vi "1D_2Period.vi"(1 "delt":dbl, 2 "1Darray":dbl[](array[numeric])) -> (0 "T2":dbl)   [LabVIEW 2020]
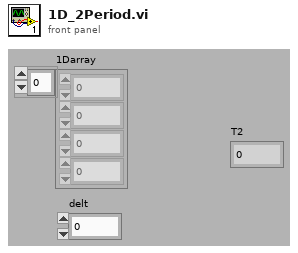
[diagram p1: front panel]
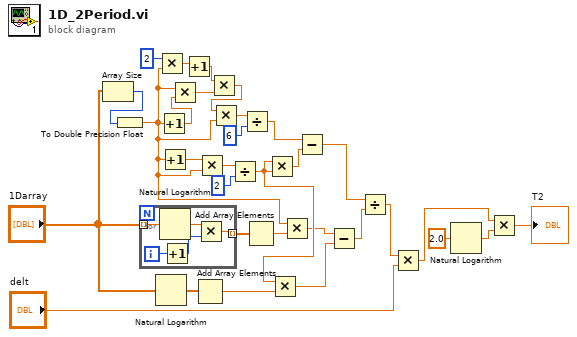
[diagram p0: block diagram]
diagram:
  n1 = Array Size(array="1Darray") -> (size(s)=w8:i32)
  n2 = To Double Precision Float(number=w8) -> (double precision float=w7:dbl)
  n3 = for {
    tunnel: "1Darray" -> [w36] mode=indexing
    tunnel: [w32] -> w21 mode=indexing
    i -> [w35]
    n4 = Natural Logarithm(1:w36) -> (0:w34:dbl)
    n5 = Increment(x=w35) -> (x+1=w33:i32)
    n6 = Multiply(x=w34, y=w33) -> (x*y=w32:dbl)
  }
  n7 = Natural Logarithm(1:"1Darray") -> (0:w16:dbl[])
  n8 = Multiply(x=2 ("count"), y=w7) -> (x*y=w28:dbl)
  n9 = Increment(x=w7) -> (x+1=w31:dbl)
  n10 = Increment(x=w7) -> (x+1=w25:dbl)
  n11 = Multiply(x=w7, y=w31) -> (x*y=w29:dbl)
  n12 = Increment(x=w28) -> (x+1=w27:dbl)
  n13 = Add Array Elements(numeric array=w16) -> (sum=w15:dbl)
  n14 = Multiply(x=w25, y=w7) -> (x*y=w24:dbl)
  n15 = Multiply(x=w27, y=w29) -> (x*y=w26:dbl)
  n16 = Multiply(x=w26, y=w7) -> (x*y=w11:dbl)
  n17 = Divide(x=w24, y=2 ("count")) -> (x/y=w19:dbl)
  n18 = Divide(x=w11, y=6 ("count")) -> (x/y=w9:dbl)
  n19 = Add Array Elements(numeric array=w21) -> (sum=w22:dbl)
  n20 = Multiply(x=w19, y=w19) -> (x*y=w20:dbl)
  n21 = Multiply(x=w19, y=w15) -> (x*y=w17:dbl)
  n22 = Multiply(x=w7, y=w22) -> (x*y=w18:dbl)
  n23 = Subtract(x=w9, y=w20) -> (x-y=w13:dbl)
  n24 = Subtract(x=w18, y=w17) -> (x-y=w14:dbl)
  n25 = Divide(x=w13, y=w14) -> (x/y=w12:dbl)
  n26 = Multiply(x=w12, y="delt") -> (x*y=w4:dbl)
  n27 = Natural Logarithm(1:sgl 2.0) -> (0:w6:sgl)
  n28 = Multiply(x=w4, y=w6) -> (x*y=→"T2":dbl)
